vi "PCIe-1760.vi"() -> ()   [LabVIEW 2020]
uses:
  <vilib>/Utility/miscctls.llb/LVPointTypeDef.ctl
  LabVIEW 2020 Toolkits/toolkits_lv2020_32bit/Synchronization.llb/SynchRefs_SetGet.ctl
  LabVIEW 2020 Toolkits/VI Server Toolkit/VI Server Libraries/VI Server_GetControl.llb/VI Server_STR_Get.vi
  LabVIEW 2020 Toolkits/VI Server Toolkit/VI Server Libraries/VI Server_Set Controls.llb/Set STR Control.vi
  LabVIEW 2020 Toolkits/VI Server Toolkit/VI Server Libraries/VI Server_SetControl.llb/VI Server_BOOL_Set.vi
  LabVIEW 2020 Toolkits/VI Server Toolkit/VI Server Toolkit LV2013.lvlib
panel:
  out "System.Message":string caption="System Message"
  in  "Help":bool
  in  "FP.Hide":bool caption="FrontPanel.Hide"
  in  "EXIT":bool
  in  "Tab.Main":enum32{"Digital I/O", "SETTINGS"}(tab)
  in  "PWM.Ch2.Period.Lo":dbl caption="Period: Lo" format="%#_g ms"
  in  "PWM.Ch2.Period.Hi":dbl caption="Period: Hi" format="%#_g ms"
  in  "PWM.Ch2.Start":bool caption="Counter.Start"
  in  "PWM.Ch1.Period.Lo":dbl caption="Period: Lo" format="%#_g ms"
  in  "PWM.Ch1.Period.Hi":dbl caption="Period: Hi" format="%#_g ms"
  in  "PWM.Ch1.Start":bool caption="Counter.Start"
  in  "Relay.DisableUpdate":bool caption="Disable Update"
  in  "Relay.Reset":bool
  in  "Relays.Resend":bool
  out "Relays.Verified":bool caption="Verified"
  in  "Relay.8":bool caption="8"
  in  "Relay.7":bool caption="7"
  in  "Relay.6":bool caption="6"
  in  "Relay.5":bool caption="5"
  in  "Relay.4":bool caption="4"
  in  "Relay.3":bool caption="3"
  in  "Relay.2":bool caption="2"
  in  "Relay.1":bool caption="1"
  out "Counter.Frequency":dbl[](array[numeric]) caption="Frequency" format="%0.3f Hz"
  in  "Counter.Method":u16(ring) caption="Function" items=["Counter", "Frequency"]
  in  "Counter.Start":bool
  out "Counter.Data":i32[](array[numeric]) caption="Counts"
  out "DI.8":bool
  out "DI.7":bool
  out "DI.6":bool
  out "DI.5":bool
  out "DI.4":bool
  out "DI.3":bool
  out "DI.2":bool
  out "DI.1":bool
  in  "DI.Line.Update":bool caption="Update:"
  in  "RelayVerify.Disable":bool
  in  "VI.WindowsTitle":string caption="Windows Title"
  in  "Cont.Measurements.CycleTime":u32 caption="Continius Measurements:\nCycleTime"
  in  "UDP.Test.String2.Send":bool
  in  "UDP.Test.String2":string caption="UDP: Test String 2"
  in  "UDP.Port.BC":u16=58433 caption="UDP: Port.BC"
  in  "UDP.Port.RT":u16=58432 caption="UDP: Port.RT"
  in  "UDP.LocalPort.Write":u16=58434 caption="UDP: Local Port.Write"
  in  "UDP.IP.Address":string="234.5.6.7" caption="UDP: IP Address"
  in  "UDP.Test.String1.Send":bool
  in  "UDP.Test.String1":string caption="UDP: Test String 1"
  in  "UDP.Responce.String.Monitor":bool
  out "UDP.ExecEng.Message.String":string caption="UDP: Execution Engine Message String"
  out "error out":errorcluster
  in  "error in":errorcluster
  # "Digital Inputs"
  # "ON"
  # "OFF"
  # "PWM Output"
  # "Channel 1"
  # "Channel 2"
  # "Channel 1"
  # "Channel 2"
  # "Ch 2"
  # "Ch 1"
  # "Relays Control"
  # "Counters Input"
  # "Multicast IP addresses must be in the 224.0.0.0 to 239.255.255.255 range."
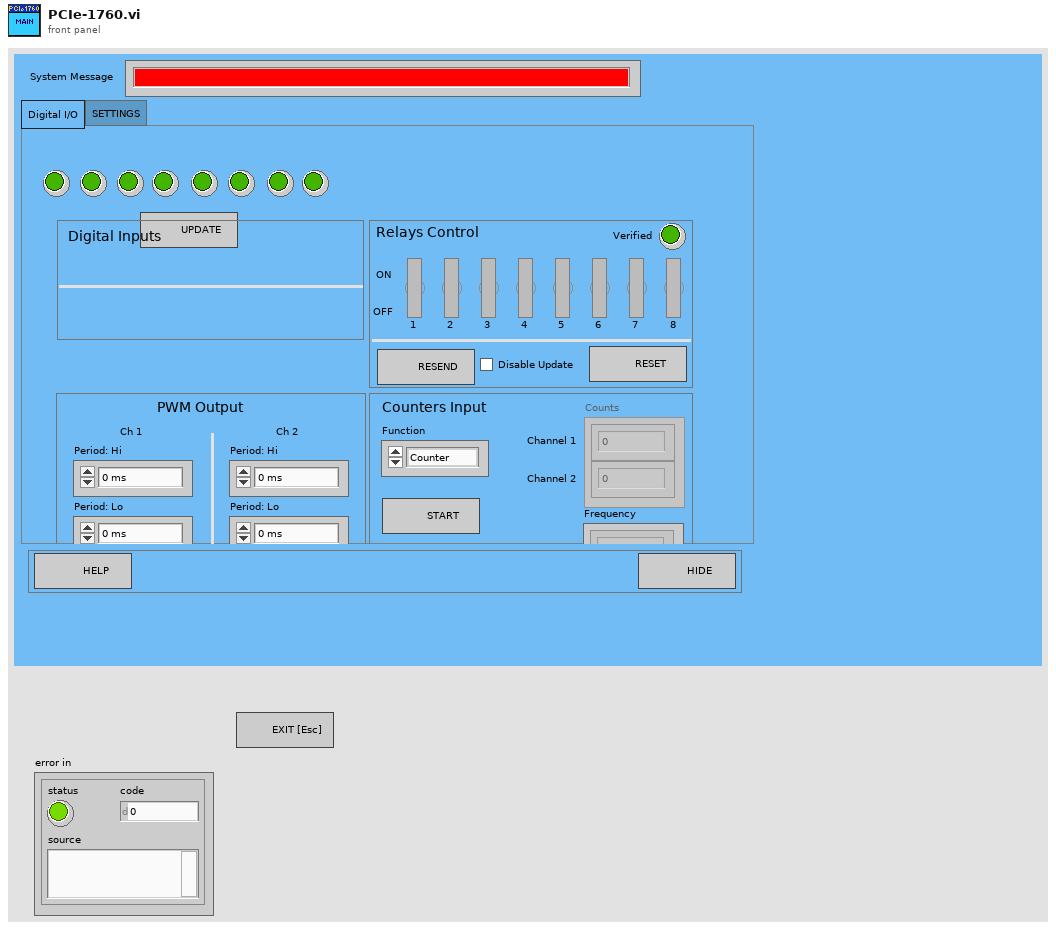
[diagram p1: front panel]
types:
  T1 = typedef "LVPointTypeDef.ctl" = cluster{"Horizontal":i16, "Vertical":i16}
  T2 = typedef "VI Server_RefsCluster.ctl" = cluster{"Labels":string[], "Refs":refnum<vi>[], "VI Ref":refnum<vi>}
  T3 = typedef "SynchRefs_SetGet.ctl" = enum16{"Set", "Get"}
  T4 = enum8{"Enabled", "Disabled", "Disabled and Grayed Out"}
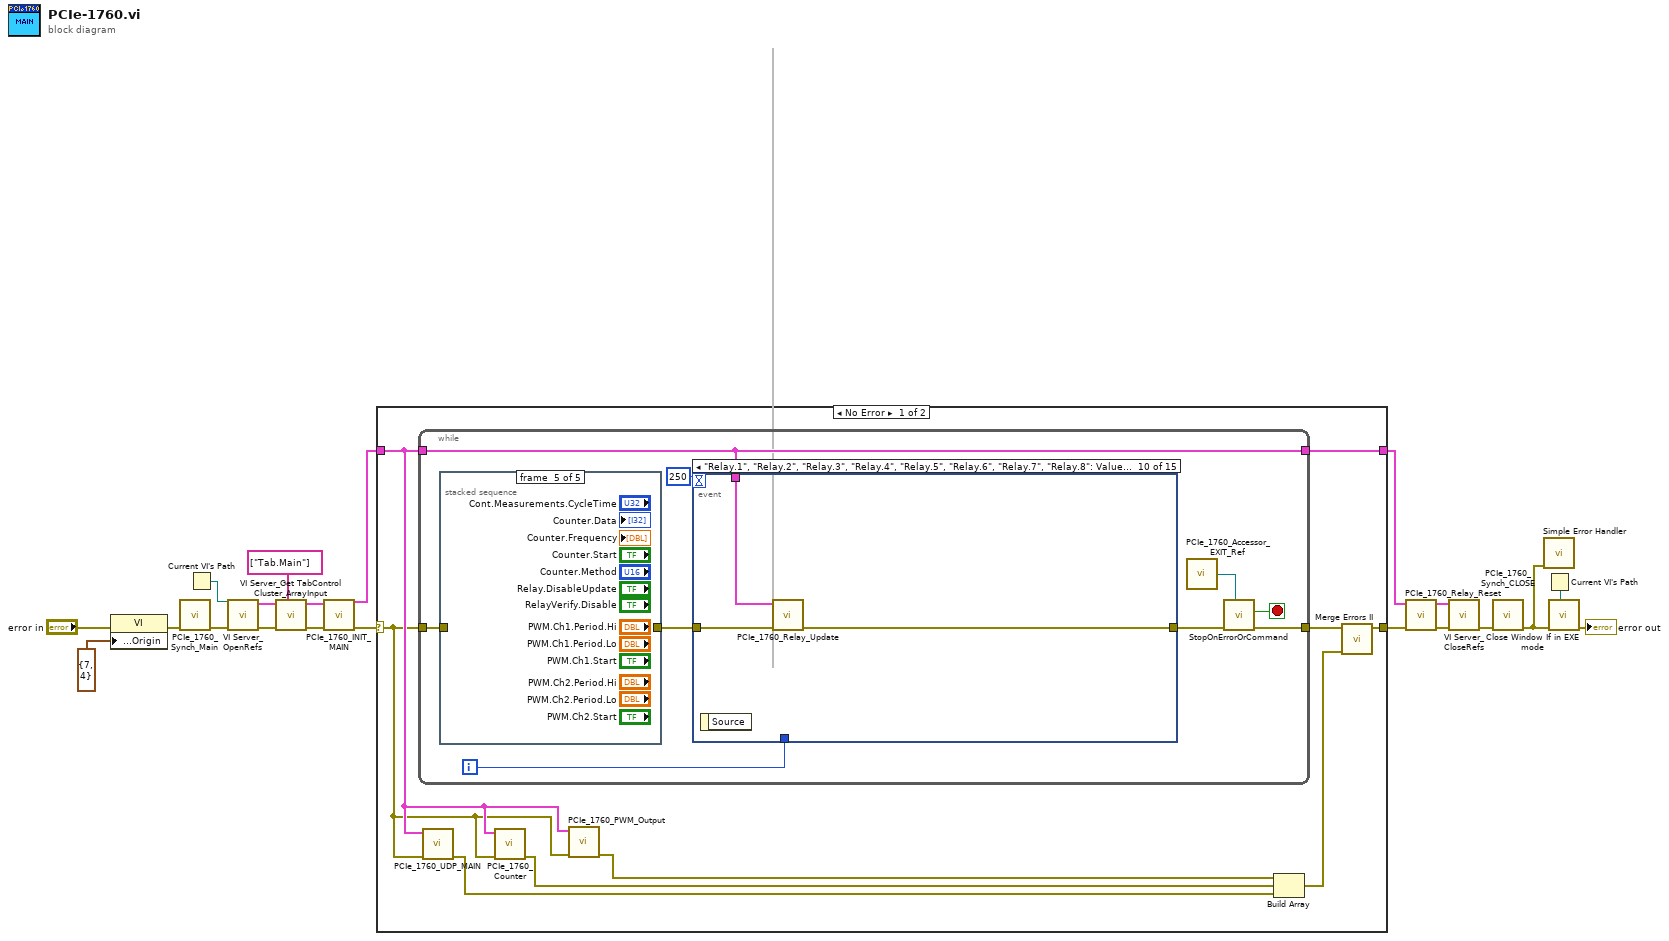
[diagram p0: block diagram]
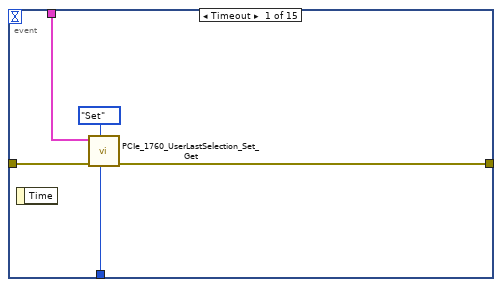
[diagram p2: hidden frame]
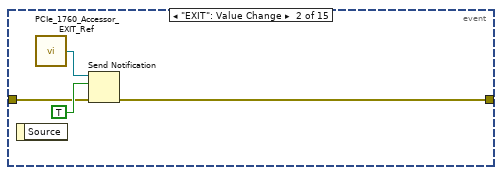
[diagram p3: hidden frame]
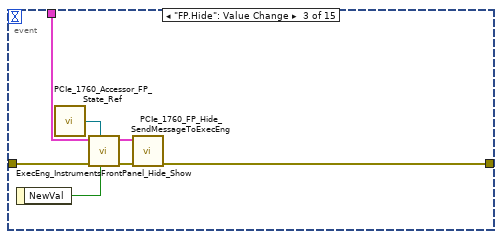
[diagram p4: hidden frame]
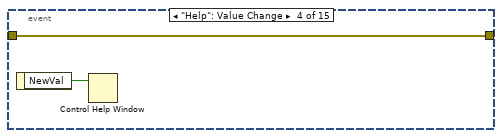
[diagram p5: hidden frame]
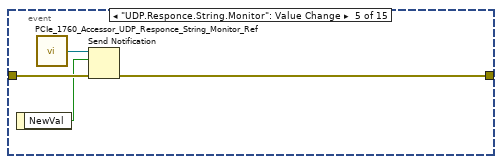
[diagram p6: hidden frame]
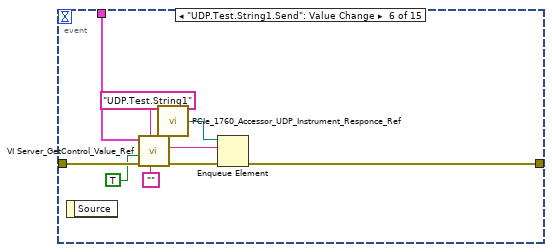
[diagram p7: hidden frame]
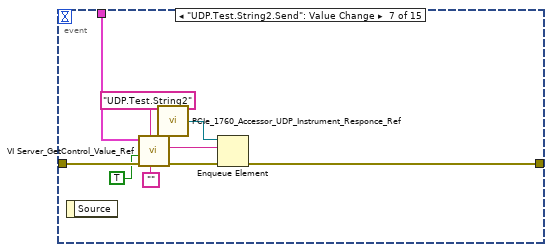
[diagram p8: hidden frame]
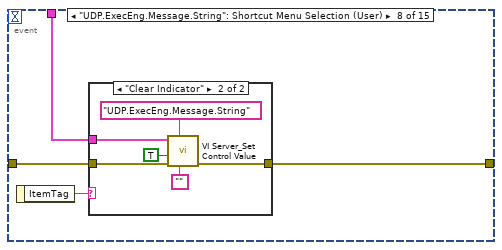
[diagram p9: hidden frame]
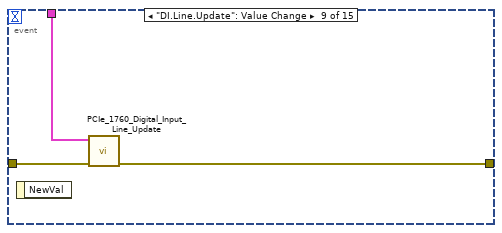
[diagram p11: hidden frame]
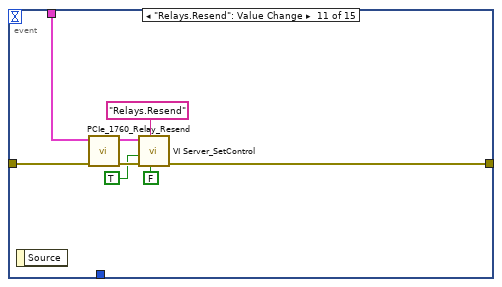
[diagram p12: hidden frame]
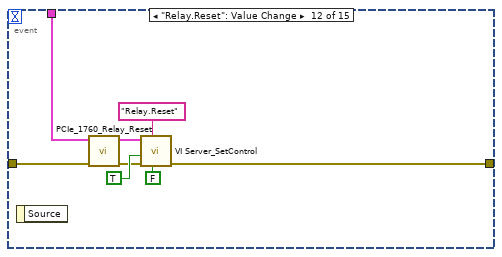
[diagram p13: hidden frame]
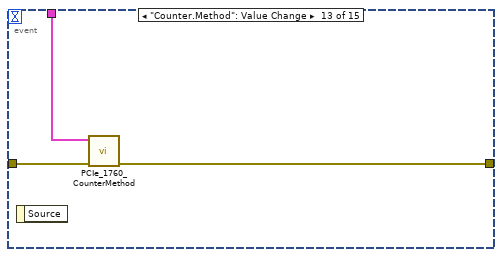
[diagram p14: hidden frame]
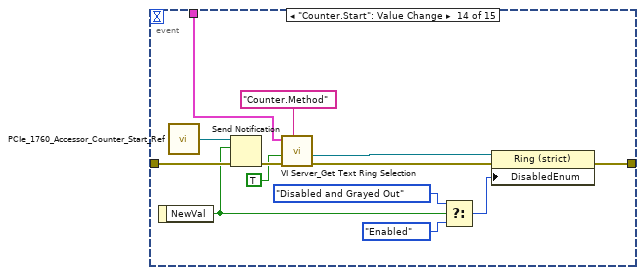
[diagram p15: hidden frame]
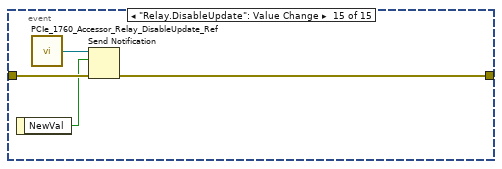
[diagram p16: hidden frame]
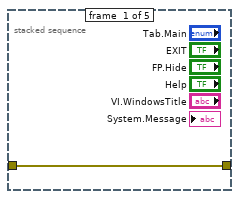
[diagram p17: hidden frame]
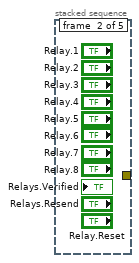
[diagram p18: hidden frame]
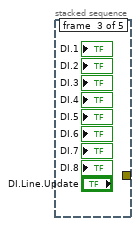
[diagram p19: hidden frame]
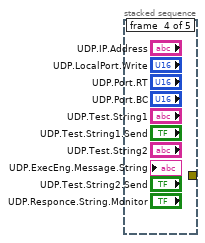
[diagram p20: hidden frame]
diagram:
  n1 = property class="VI"(error in="error in", "Front Panel Window:Origin"=T1 {"Horizontal"=7, "Vertical"=4}) -> (error out=w14:errorcluster)  [unwired: 1 in, 1 out]
  n2 = call "PCIe_1760_Synch_Main.vi"("error in"=w14) -> ("error out"=w15:errorcluster)  [unwired: 10 in]
  n3 = Current VI's Path() -> (path=w19:path)
  n4 = call "VI Server_OpenRefs.vi"("error in"=w15, "VI Path"=w19) -> ("error out"=w16:errorcluster, "VI Server.RefsCluster"=w17:T2)  [unwired: 8 in]
  n5 = call "VI Server_Get TabControl Cluster_ArrayInput.vi"("TabControl Labels[]"=string[] ["Tab.Main"], "error in"=w16, "VI Server Cluster"=w17) -> ("error out"=w13:errorcluster, "VI Server Cluster.OUT"=w12:T2)  [unwired: 7 in]
  n6 = call "PCIe_1760_INIT_MAIN.vi"("error in (no error)"=w13, "VI Server Cluster"=w12) -> ("error out"=w11:errorcluster, "VI Server Cluster DUP"=w10:T2)  [unwired: 8 in]
  n7 = case shown="No Error" w11 {
    selector: w11 -> [w22 w134]
    tunnel: [w26 w134] -> w6
    tunnel: w10 -> [w23 w133]
    tunnel: [w29 w133] -> w3
    frame No Error {
      n8 = while {
        tunnel: w22 -> [w38]
        tunnel: [w32] -> w27
        tunnel: w23 -> [w34]
        tunnel: [w34] -> w29
        i -> [w35]
        stop <- w31 stop-if-true
        n9 = stacked-sequence {
          tunnel: w38 -> [w132 _ _ _ _]
          tunnel: [w132 _ _ _ _] -> w37
          frame #0 {
          }
          frame #1 {
          }
          frame #2 {
          }
          frame #3 {
          }
          frame #4 {
          }
        }
        n10 = event shown="[9] \"Relay.1\", \"Relay.2\", \"Relay.3\", \"Relay.4\", \"Relay.5\", \"Relay.6\", \"Relay.7\", \"Relay.8\": Value Change" {
          selector: _ -> [_ _ _ _ _ _ _ _ _ _ _ _ _ _ _]
          dyn-events: _ -> [_ _ _ _ _ _ _ _ _ _ _ _ _ _ _]
          timeout: 250 -> [_ _ _ _ _ _ _ _ _ _ _ _ _ _ _]
          tunnel: w37 -> [w42 w44 w53 w56 w60 w69 w78 w82 w92 w94 w102 w111 w114 w127 w131]
          tunnel: w35 -> [w41 _ _ _ _ _ _ _ _ _ _ _ _ _ _]
          tunnel: [w39 w46 w54 w56 w58 w67 w76 w80 w91 w93 w100 w106 w112 w120 w130] -> w33
          tunnel: w34 -> [w40 _ w50 _ _ w66 w75 w79 w90 w95 w103 w110 w113 w123 _]
          event Timeout {
            n11 = event-data() -> ()  [unwired: 1 in, 1 out]
            n12 = call "PCIe_1760_UserLastSelection_Set_Get.vi"("LoopCounter"=w41, "SynchRefs.Set/Get"=SynchRefs_SetGet."Set", "error in"=w42, "VI Server.RefsCluster"=w40) -> ("error out"=w39:errorcluster)  [unwired: 6 in, 1 out]
          }
          event "EXIT": Value Change {
            n13 = event-data() -> ()  [unwired: 1 in, 1 out]
            n14 = call "PCIe_1760_Accessor_EXIT_Ref.vi"() -> ("EXIT"=w47:refnum<notifier>)  [unwired: 6 in]
            n15 = Send Notification(notification=TRUE, notifier=w47, error in (no error)=w44) -> (error out=w46:errorcluster)  [unwired: 1 out]
          }
          event "FP.Hide": Value Change {
            n16 = event-data() -> ("NewVal"=w51:bool)  [unwired: 1 in]
            n17 = call "PCIe_1760_Accessor_FP_State_Ref.vi"() -> ("FP.State"=w48:refnum<notifier>)  [unwired: 6 in]
            n18 = call "ExecEng_InstrumentsFrontPanel_Hide_Show.vi"("FP.Hide/Show"=w51, "FP.State"=w48, "error in (no error)"=w53, "VI Server Cluster"=w50) -> ("error out"=w52:errorcluster, "VI Server Cluster DUP"=w49:T2)  [unwired: 6 in]
            n19 = call "PCIe_1760_FP_Hide_SendMessageToExecEng.vi"("error in (no error)"=w52, "VI Server Cluster"=w49) -> ("error out"=w54:errorcluster)  [unwired: 9 in]
          }
          event "Help": Value Change {
            n20 = event-data() -> ("NewVal"=w55:bool)  [unwired: 1 in]
            n21 = Control Help Window(1:w55) -> ()  [unwired: 1 in]
          }
          event "UDP.Responce.String.Monitor": Value Change {
            n22 = event-data() -> ("NewVal"=w57:bool)  [unwired: 1 in]
            n23 = call "PCIe_1760_Accessor_UDP_Responce_String_Monitor_Ref.vi"() -> ("UDP.ExecEng.Command.String.Monitor"=w59:refnum<notifier>)  [unwired: 6 in]
            n24 = Send Notification(notification=w57, notifier=w59, error in (no error)=w60) -> (error out=w58:errorcluster)  [unwired: 1 out]
          }
          event "UDP.Test.String1.Send": Value Change {
            n25 = event-data() -> ()  [unwired: 1 in, 1 out]
            n26 = call-poly "VI Server_GetControl_Value_Ref.vi"("DataType"="", "Control.Label"="UDP.Test.String1", "error in"=w69, "SingleInstance"=TRUE, "VI Server.RefsCluster"=w66) -> ("error out"=w68:errorcluster, "Value"=w61:string)  [unwired: 3 in, 2 out]
            n27 = call "PCIe_1760_Accessor_UDP_Instrument_Responce_Ref.vi"() -> ("UDP.Instrument.Responce.Q"=w62:refnum<queue>)  [unwired: 6 in]
            n28 = Enqueue Element(queue=w62, element=w61, error in (no error)=w68) -> (error out=w67:errorcluster)  [unwired: 1 in, 2 out]
          }
          event "UDP.Test.String2.Send": Value Change {
            n29 = event-data() -> ()  [unwired: 1 in, 1 out]
            n30 = call-poly "VI Server_GetControl_Value_Ref.vi"("DataType"="", "Control.Label"="UDP.Test.String2", "error in"=w78, "SingleInstance"=TRUE, "VI Server.RefsCluster"=w75) -> ("error out"=w77:errorcluster, "Value"=w70:string)  [unwired: 3 in, 2 out]
            n31 = call "PCIe_1760_Accessor_UDP_Instrument_Responce_Ref.vi"() -> ("UDP.Instrument.Responce.Q"=w71:refnum<queue>)  [unwired: 6 in]
            n32 = Enqueue Element(queue=w71, element=w70, error in (no error)=w77) -> (error out=w76:errorcluster)  [unwired: 1 in, 2 out]
          }
          event "UDP.ExecEng.Message.String": Shortcut Menu Selection (User) {
            n33 = event-data() -> ("ItemTag"=w81:string)  [unwired: 1 in]
            n34 = case shown="\"Clear Indicator\"" w81 {
              tunnel: w82 -> [w83 w89]
              tunnel: [w83 w88] -> w80
              tunnel: w79 -> [_ w87]
              frame "", Default {
              }
              frame "Clear Indicator" {
                n35 = call-poly "VI Server_Set Control Value.vi"("New Value"="", "Label"="UDP.ExecEng.Message.String" ("Control.Label"), "error in"=w89, "Single Instance (T)"=TRUE ("SingleInstance"), "VI Server Cluster"=w87) -> ("error out"=w88:errorcluster)  [unwired: 4 in, 2 out]
              }
            }
          }
          event "DI.Line.Update": Value Change {
            n36 = event-data() -> ()  [unwired: 1 in, 1 out]
            n37 = call "PCIe_1760_Digital_Input_Line_Update.vi"("error in (no error)"=w92, "VI Server Cluster"=w90) -> ("error out"=w91:errorcluster)  [unwired: 9 in]
          }
          event "Relay.1", "Relay.2", "Relay.3", "Relay.4", "Relay.5", "Relay.6", "Relay.7", "Relay.8": Value Change {
            n38 = event-data() -> ()  [unwired: 1 in, 1 out]
            n39 = call "PCIe_1760_Relay_Update.vi"("error in (no error)"=w94, "VI Server Cluster"=w95) -> ("error out"=w93:errorcluster)  [unwired: 8 in, 1 out]
          }
          event "Relays.Resend": Value Change {
            n40 = event-data() -> ()  [unwired: 1 in, 1 out]
            n41 = call "PCIe_1760_Relay_Resend.vi"("error in (no error)"=w102, "VI Server Cluster"=w103) -> ("error out"=w101:errorcluster, "VI Server Cluster.DUP"=w99:T2)  [unwired: 8 in]
            n42 = call-poly "VI Server_SetControl.vi"("Data"=FALSE, "Control.Label"="Relays.Resend", "error in"=w101, "SingleInstance"=TRUE, "VI Server.RefsCluster"=w99) -> ("error out"=w100:errorcluster)  [unwired: 4 in, 2 out]
          }
          event "Relay.Reset": Value Change {
            n43 = event-data() -> ()  [unwired: 1 in, 1 out]
            n44 = call "PCIe_1760_Relay_Reset.vi"("error in (no error)"=w111, "VI Server Cluster"=w110) -> ("error out"=w107:errorcluster, "VI Server Cluster.DUP"=w104:T2)  [unwired: 7 in, 1 out]
            n45 = call-poly "VI Server_SetControl.vi"("Data"=FALSE, "Control.Label"="Relay.Reset", "error in"=w107, "SingleInstance"=TRUE, "VI Server.RefsCluster"=w104) -> ("error out"=w106:errorcluster)  [unwired: 4 in, 2 out]
          }
          event "Counter.Method": Value Change {
            n46 = event-data() -> ()  [unwired: 1 in, 1 out]
            n47 = call "PCIe_1760_CounterMethod.vi"("error in (no error)"=w114, "VI Server Cluster"=w113) -> ("error out"=w112:errorcluster)  [unwired: 8 in, 1 out]
          }
          event "Counter.Start": Value Change {
            n48 = event-data() -> ("NewVal"=w117:bool)  [unwired: 1 in]
            n49 = call "PCIe_1760_Accessor_Counter_Start_Ref.vi"() -> ("Counter.Start"=w126:refnum<notifier>)  [unwired: 6 in]
            n50 = Send Notification(notification=w117, notifier=w126, error in (no error)=w127) -> (error out=w125:errorcluster)  [unwired: 1 out]
            n51 = call "VI Server_Get Text Ring Selection.vi"("Label"="Counter.Method", "error in"=w125, "Single Instance (T)"=TRUE, "VI Server Cluster"=w123) -> ("error out"=w121:errorcluster, "Control Reference"=w119:refnum<vi>)  [unwired: 2 in, 4 out]
            n52 = Select(t=T4."Disabled and Grayed Out", s=w117, f=T4."Enabled" ("Disabled")) -> (s? t:f=w116:T4)
            n53 = property class="Ring (strict)"(reference=w119, error in=w121, "DisabledEnum"=w116) -> (error out=w120:errorcluster)  [unwired: 1 out]
          }
          event "Relay.DisableUpdate": Value Change {
            n54 = event-data() -> ("NewVal"=w129:bool)  [unwired: 1 in]
            n55 = call "PCIe_1760_Accessor_Relay_DisableUpdate_Ref.vi"() -> ("Relay.DisableUpdate"=w128:refnum<notifier>)  [unwired: 6 in]
            n56 = Send Notification(notification=w129, notifier=w128, error in (no error)=w131) -> (error out=w130:errorcluster)  [unwired: 1 out]
          }
        }
        n57 = call "PCIe_1760_Accessor_EXIT_Ref.vi"() -> ("EXIT"=w30:refnum<notifier>)  [unwired: 6 in]
        n58 = call "StopOnErrorOrCommand.vi"("STOP"=w30, "error in (no error)"=w33) -> ("error out"=w32:errorcluster, "STOP"=w31:bool)  [unwired: 8 in]
      }
      n59 = call "PCIe_1760_UDP_MAIN.vi"("error in (no error)"=w22, "VI Server.RefsCluster"=w23) -> ("error out"=w28:errorcluster)  [unwired: 9 in]
      n60 = call "PCIe_1760_Counter.vi"("error in (no error)"=w22, "VI Server Cluster"=w23) -> ("error out"=w24:errorcluster)  [unwired: 9 in]
      n61 = call "PCIe_1760_PWM_Output.vi"("error in (no error)"=w22, "VI Server Cluster"=w23) -> ("error out"=w21:errorcluster)  [unwired: 9 in]
      n62 = Build Array(w21, w24, w28) -> (w25:errorcluster[])
      n63 = call "Merge Errors II.vi"("error array in"=w25, "error in 1 (no error)"=w27) -> ("error out.DUP"=w26:errorcluster)  [unwired: 4 in, 1 out]
    }
    frame Error {
    }
  }
  n64 = call "PCIe_1760_Relay_Reset.vi"("error in (no error)"=w6, "VI Server Cluster"=w3) -> ("error out"=w5:errorcluster, "VI Server Cluster.DUP"=w4:T2)  [unwired: 7 in, 1 out]
  n65 = call "VI Server_CloseRefs.vi"("error in"=w5, "VI Server.RefsCluster"=w4) -> ("error out"=w9:errorcluster)  [unwired: 9 in]
  n66 = call "PCIe_1760_Synch_CLOSE.vi"("error in"=w9) -> ("error out"=w2:errorcluster)  [unwired: 10 in]
  n67 = call <vilib>:"Simple Error Handler.vi"("error in (no error)"=w2) -> ()  [unwired: 4 in, 5 out]
  n68 = Current VI's Path() -> (path=w1:path)
  n69 = call "Close Window If in EXE mode.vi"("TopLevelVI Path"=w1, "error in"=w2) -> ("error out"=→"error out":errorcluster)  [unwired: 9 in]
